vi "Get Attribute as JSON.vi"(8 "error in":errorcluster, 10 "Attribute":string, 11 "Config from XML in":refnum<class "Config from XML.lvclass">) -> (0 "error out":errorcluster, 2 "<JSON>":string, 3 "Config from XML out":refnum<class "Config from XML.lvclass">)   [LabVIEW 2025, in "Config from XML.lvclass"]
uses:
  Config from XML.lvclass
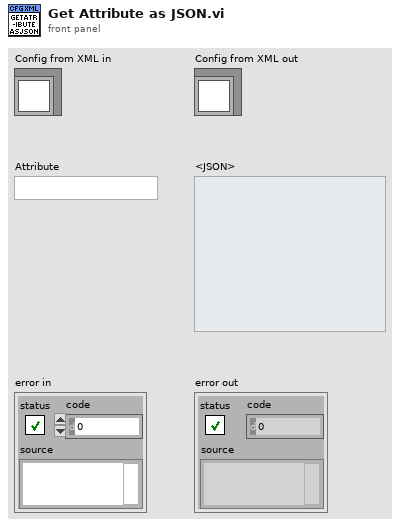
[diagram p1: front panel]
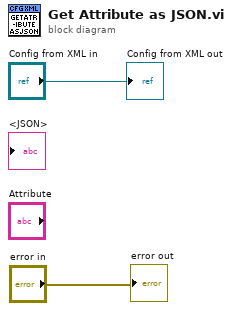
[diagram p0: block diagram]
diagram:
  "error out" <- "error in"
  "Config from XML out" <- "Config from XML in"
